vi "Hitrap_DiagnosticBoxGUI.contents.vi"   [LabVIEW 2014, in "Hitrap_DiagnosticBoxGUI.lvlib"]
uses:
  Hitrap_DiagnosticBoxGUI.lvlib
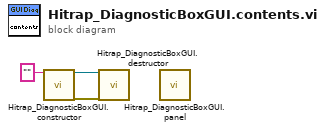
[diagram p0: block diagram]
diagram:
  n1 = call "Hitrap_DiagnosticBoxGUI.constructor.vi"("name"="") -> ("i ref out"=w2:refnum<vi>, "error out"=w1:errorcluster)  [unwired: 16 in, 1 out]
  n2 = call "Hitrap_DiagnosticBoxGUI.destructor.vi"("i ref in"=w2, "error in (no error)"=w1) -> ()  [unwired: 17 in, 1 out]
  n3 = call "Hitrap_DiagnosticBoxGUI.panel.vi"() -> ()  [unwired: 1 in]
